vi "固定点.vi"(2 "DY":dbl, 3 "DX":dbl, 4 "TY":dbl, 5 "TX":dbl, 6 "HY":dbl, 7 "HX":dbl) -> (0 "R":i16, 1 "L":i16)   [LabVIEW 2013]
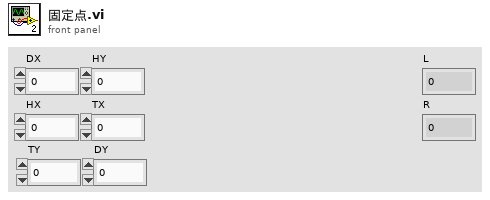
[diagram p1: front panel]
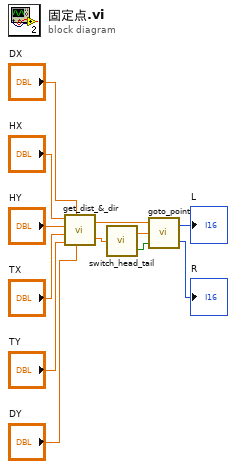
[diagram p0: block diagram]
diagram:
  n1 = call "get_dist_&_dir.vi"("DY"="DY", "DX"="DX", "TY"="TY", "TX"="TX", "HY"="HY", "HX"="HX") -> ("direction"=w12:dbl, "distance"=w11:dbl)
  n2 = call "switch_head_tail.vi"("del_in"=w12) -> ("del_out"=w9:dbl, "rev?"=w10:bool)
  n3 = call "goto_point.vi"("rev"=w10, "direction"=w9, "distance"=w11) -> ("R"=→"R":i16, "L"=→"L":i16)
